vi "Stop Channel.vi"(8 "error in (no error)":errorcluster, 9 "ChannelType":enum16{"Device", "Ch0", "Ch1"}(ring), 11 "DevState":T1={"Type"=41, "Index"=0, "DeviceOpen"=FALSE, "Ch0Start"=FALSE, "Ch1Start"=FALSE} {"Index" items=["0", "1", "2", "3", "4", "5", "6", "7", "8"]; "Type" items=["USBCANFD-200U"=41, "USBCANFD-100U"=42]}) -> (0 "error out":errorcluster, 3 "DevState out":T1={"Type"=41, "Index"=0, "DeviceOpen"=FALSE, "Ch0Start"=FALSE, "Ch1Start"=FALSE} {"Index" items=["0", "1", "2", "3", "4", "5", "6", "7", "8"]; "Type" items=["USBCANFD-200U"=41, "USBCANFD-100U"=42]})   [LabVIEW 2018, in "CAN FD.lvlib"]
uses:
  CAN FD.lvlib
  SubVI/zlgcan.lvlib
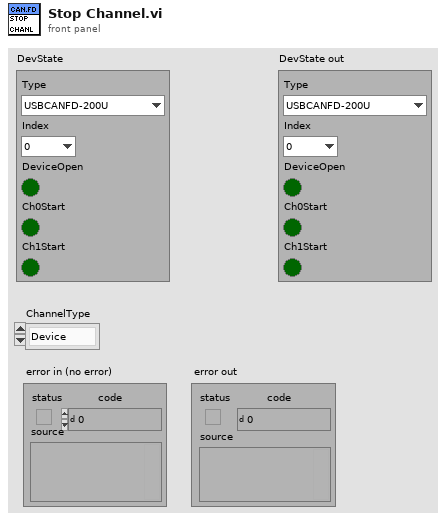
[diagram p1: front panel]
types:
  T1 = cluster{"Type":u32, "Index":u32, "DeviceOpen":bool, "Ch0Start":bool, "Ch1Start":bool}
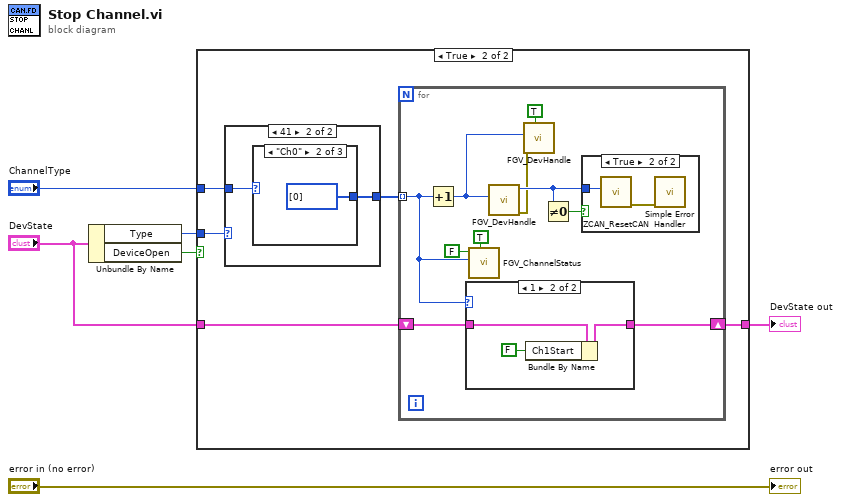
[diagram p0: block diagram]
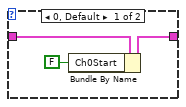
[diagram p3: hidden frame]
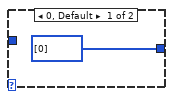
[diagram p5: hidden frame]
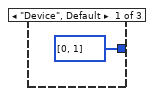
[diagram p6: hidden frame]
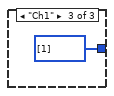
[diagram p7: hidden frame]
diagram:
  n1 = Unbundle By Name("DevState") -> ("Type"=w3:u32, "DeviceOpen"=w6:bool)
  n2 = case shown="True" w6 {
    tunnel: "ChannelType" -> [_ w11]
    tunnel: w3 -> [_ w12]
    tunnel: "DevState" -> [w7 w9]
    tunnel: [w7 w8] -> w1
    frame False {
    }
    frame True {
      n3 = case shown="41" w12 {
        tunnel: w11 -> [_ w33]
        tunnel: [i32[] [0] w32] -> w10
        frame 0, Default {
        }
        frame 41 {
          n4 = case shown="\"Ch0\"" w33 {
            tunnel: [i32[] [0, 1] i32[] [0] i32[] [1]] -> w32
            frame "Device", Default {
            }
            frame "Ch0" {
            }
            frame "Ch1" {
            }
          }
        }
      }
      n5 = for {
        tunnel: w10 -> [w18] mode=indexing
        shift-right: [w19] -> w8
        shift-left: w9 -> [w20]
        n6 = Increment(x=w18) -> (x+1=w14:i32)
        n7 = case shown="1" w18 {
          tunnel: w20 -> [w25 w28]
          tunnel: [w23 w26] -> w19
          frame 0, Default {
            n8 = Bundle By Name(cluster=w25, "Ch0Start"=FALSE) -> (w23:T1)
          }
          frame 1 {
            n9 = Bundle By Name(cluster=w28, "Ch1Start"=FALSE ("Ch0Start")) -> (w26:T1)
          }
        }
        n10 = call "FGV_ChannelStatus.vi"("Set"=TRUE, "Index"=w18, "Start"=FALSE) -> ()  [unwired: 7 in, 2 out]
        n11 = call "FGV_DevHandle.vi"("Type"=w14) -> ("error out"=w15:errorcluster, "handle out"=w21:u64)  [unwired: 8 in, 1 out]
        n12 = call "FGV_DevHandle.vi"("Set"=TRUE, "error in (no error)"=w15, "Type"=w14) -> ()  [unwired: 6 in, 3 out]
        n13 = Not Equal To 0?(x=w21) -> (x != 0?=w22:bool)
        n14 = case shown="True" w22 {
          tunnel: w21 -> [_ w30]
          frame False {
          }
          frame True {
            n15 = call "ZCAN_ResetCAN.vi"("can_handle"=w30) -> ("error out"=w29:errorcluster)  [unwired: 9 in, 1 out]
            n16 = call <vilib>:"Simple Error Handler.vi"("error in (no error)"=w29) -> ()  [unwired: 4 in, 5 out]
          }
        }
      }
    }
  }
  "DevState out" <- w1
  "error out" <- "error in (no error)"
